vi "Initialize.vi"(8 "error in (no error)":errorcluster, 11 "SS P100 Settings":T1) -> (0 "error out":errorcluster, 2 "Connection Error":bool, 3 "SS P100 Settings":T1)   [LabVIEW 2018, in "Sonic Systems P100.lvlib"]
uses:
  Sonic Systems P100.lvlib
  Sonic Systems P100 Settings.ctl
  <vilib>/Instr/_visa.llb/VISA Configure Serial Port (Instr).vi
  support/Support Library.lvlib
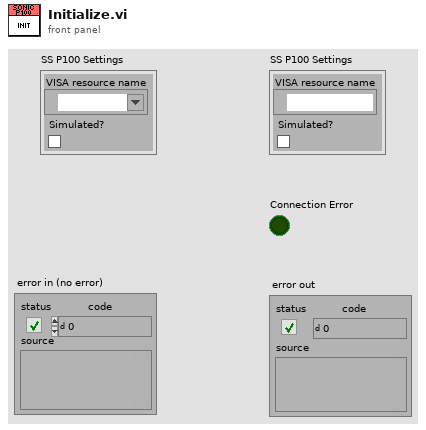
[diagram p1: front panel]
types:
  T1 = typedef "Sonic Systems P100.lvlib/Sonic Systems P100 Settings.ctl" = cluster{"VISA resource name":refnum<visa-resource-name>, "Simulated?":bool}
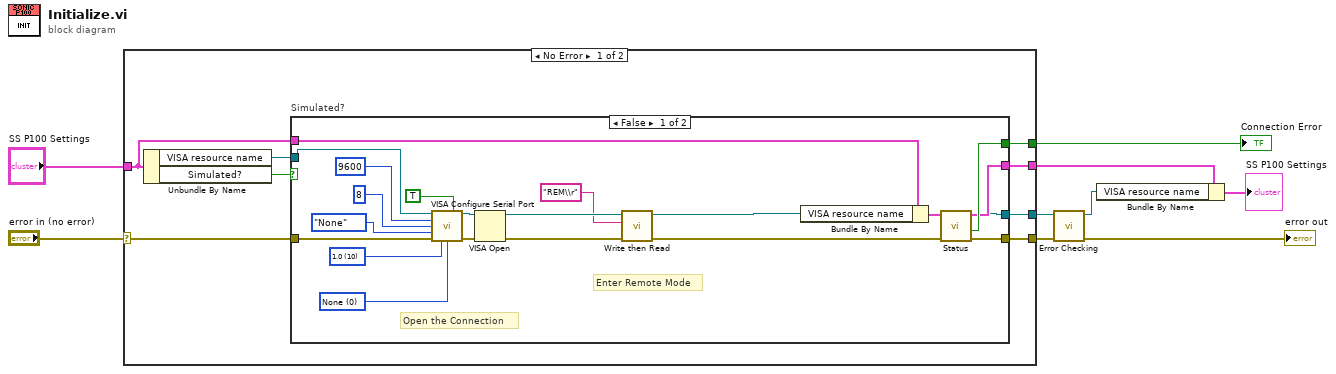
[diagram p0: block diagram]
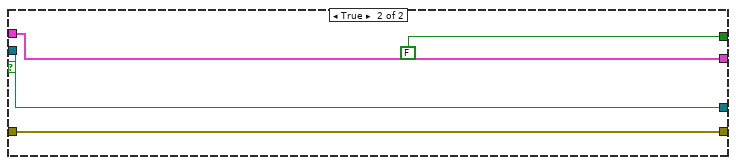
[diagram p2: hidden frame]
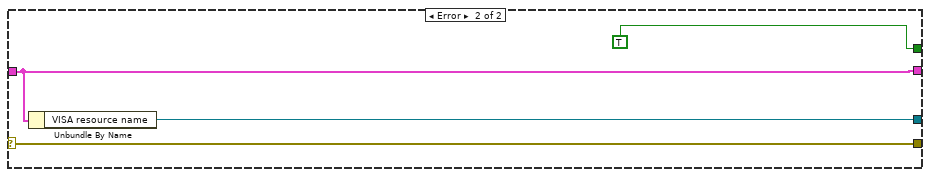
[diagram p3: hidden frame]
diagram:
  n1 = case shown="No Error" "error in (no error)" {
    selector: "error in (no error)" -> [w17 w45]
    tunnel: "SS P100 Settings" -> [w11 w42]
    tunnel: [w16 w45] -> w7
    tunnel: [w14 w44] -> w8
    tunnel: [w12 TRUE] -> w4
    tunnel: [w10 w42] -> w3
    frame No Error {
      n2 = Unbundle By Name(w11) -> ("VISA resource name"=w15:refnum<visa-resource-name>, "Simulated?"=w13:bool)
      n3 = case "Simulated?" shown="False" w13 {
        tunnel: w17 -> [w31 w41]
        tunnel: [w23 w41] -> w16
        tunnel: [w20 w40] -> w14
        tunnel: w15 -> [w29 w40]
        tunnel: [w25 FALSE] -> w12
        tunnel: w11 -> [w27 w38]
        tunnel: [w24 w38] -> w10
        frame False {
          w33 = u16 0 items=["None", "XON/XOFF", "RTS/CTS", "XON/XOFF & RTS/CTS", "DTR/DSR", "XON/XOFF & DTR/DSR"] ("flow control (0:none)")
          w34 = u16 10 items=["1.0"=10, "1.5"=15, "2.0"=20] ("stop bits (10: 1 bit)")
          # "Enter Remote Mode"
          # "Open the Connection"
          n4 = call-poly "VISA Configure Serial Port"("VISA resource name"=w29, "Enable Termination\nChar (T)"=TRUE ("Enable Termination\nChar (T)"), "baud rate (9600)"=u32 9600, "data bits (8)"=u16 8, "parity (0:none)"=enum16{"None", "Odd", "Even", "Mark", "Space"}."None", "error in (no error)"=w31, "stop bits (10: 1 bit)"=w34, "flow control (0:none)"=w33) -> ("VISA resource name out"=w30:refnum<visa-resource-name>, "error out"=w32:errorcluster)  [unwired: 6 in]
          n5 = VISA Open(error in (no error)=w32, VISA resource name=w30) -> (VISA resource name=w22:refnum<visa-resource-name>, error out=w21:errorcluster)  [unwired: 3 in]
          n6 = call "Write then Read.vi"("error in"=w21, "write buffer"="REM\\r", "VISA resource name in"=w22) -> ("error out"=w19:errorcluster, "VISA resource name out"=w20:refnum<visa-resource-name>)  [unwired: 6 in, 1 out]
          n7 = Bundle By Name(cluster=w27, "VISA resource name"=w20) -> (w26:T1)
          n8 = call "Status.vi"("error in (no error)"=w19, "SS P100 Settings In"=w26) -> ("error out"=w23:errorcluster, "Connection Error"=w25:bool, "SS P100 Settings Out"=w24:T1)  [unwired: 4 in, 3 out]
        }
        frame True {
        }
      }
    }
    frame Error {
      n9 = Unbundle By Name(w42) -> ("VISA resource name"=w44:refnum<visa-resource-name>)
    }
  }
  "Connection Error" <- w4
  n10 = call "Error Checking.vi"("error in (no error)"=w7, "VISA resource name"=w8) -> ("error out"=→"error out":errorcluster, "VISA resource name"=w5:refnum<visa-resource-name>)  [unwired: 7 in, 1 out]
  n11 = Bundle By Name(cluster=w3, "VISA resource name"=w5) -> (→"SS P100 Settings":T1)
